vi "Display.vi"(8 "error in":errorcluster, 11 "Plain Parent in":refnum<class "Plain Parent.lvclass">) -> (0 "error out":errorcluster, 3 "Plain Parent out":refnum<class "Plain Parent.lvclass">)   [LabVIEW 2021, in "Pop-Up.lvlib" / "Plain Parent.lvclass"]
doc: "This is the override method required for each child of the pop up class. It is the pop up that will display to the user.\n\nTo extend this function, create a child class of the pop up class. Then create an override method for this VI. <b>Display.vi</b> is a protected function, therefore it cannot be called in a main application. This VI must be called by a caller function. See one of the standard pop-ups for a setup example.\n\n<b>Code Developed By:</b> +\nDaniel Coons +\nhttps://github.com/danielcoons/tsc-pop-up"
uses:
  Plain Parent.lvclass
  Popup/Popup.lvclass
  Plain Parent.lvclass/Plain Parent.ctl
panel:
  # "This VI displays the popup"
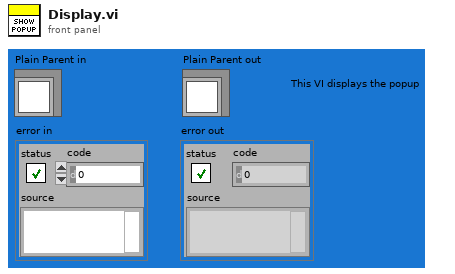
[diagram p1: front panel]
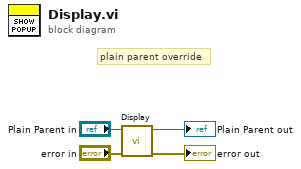
[diagram p0: block diagram]
diagram:
  # "plain parent override"
  n1 = call-parent "Display.vi"("error in"="error in", "Popup in"="Plain Parent in") -> ("error out"=→"error out":errorcluster, "Popup out"=→"Plain Parent out":refnum<class "Plain Parent.lvclass">)  [unwired: 8 in]
